vi "Email_With_Log.vi"(0 "recipients":string[](array[string]), 1 "subject ([No Subject])":string="[No Subject]", 2 "message":string, 3 "attachments":T1(array[cluster])) -> (5 "invalid recipients":string[](array[string]), 6 "error out":errorcluster)   [LabVIEW 2016]
uses:
  Globals/Preference_global.vi
  Globals/Constants_global.vi
  <vilib>/Utility/SMTP/NI_SMTPEmail.lvlib
panel:
  out "Number of valid email requests":i32
  # "Image/x-png"
  # "Image/jpeg"
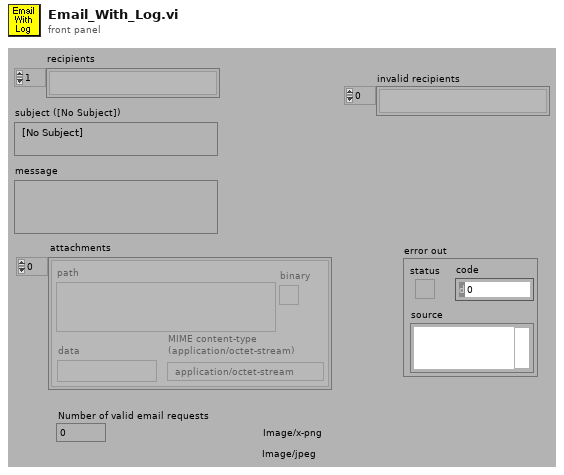
[diagram p1: front panel]
types:
  T1 = cluster{"path":path, "data":string, "binary":bool, "MIME content-type \n(application/octet-stream)":string}[]
  T2 = cluster{"path":path, "data":string, "binary":bool, "MIME content-type \n(application/octet-stream)":string}
  T3 = typedef "SMTPCredentials.ctl" = cluster{"User Name":string, "Password":string, "Reply to Address":string, "From Domain":string}
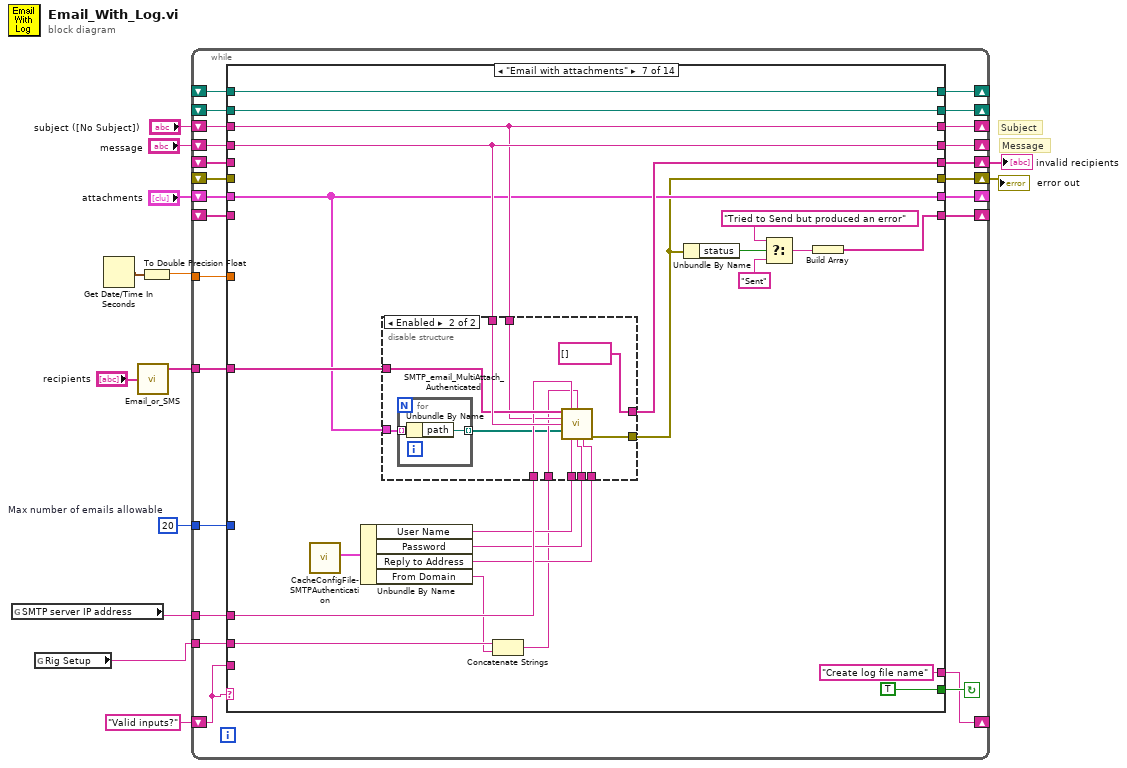
[diagram p0: block diagram]
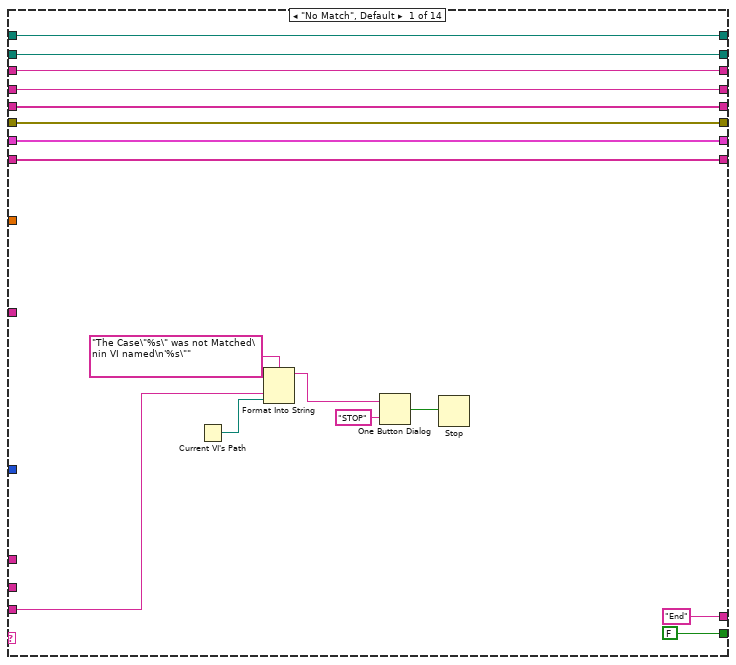
[diagram p2: hidden frame]
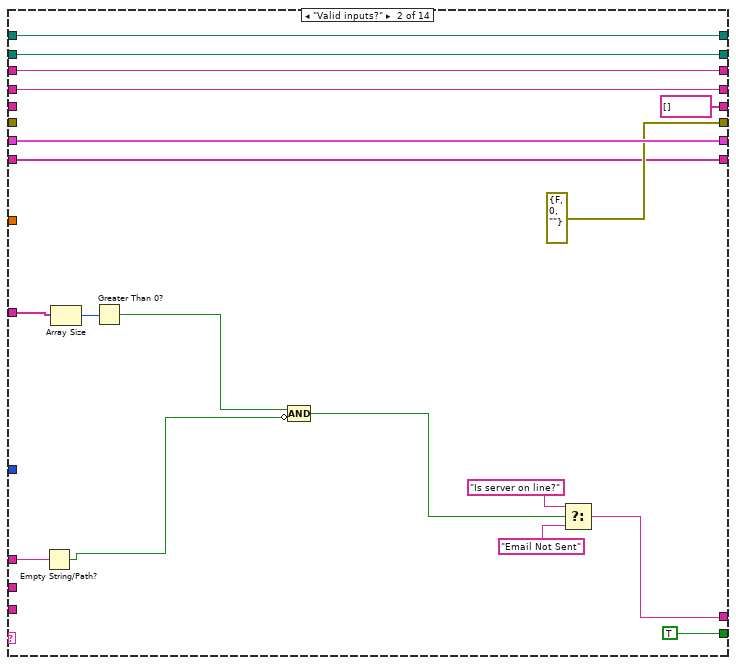
[diagram p3: hidden frame]
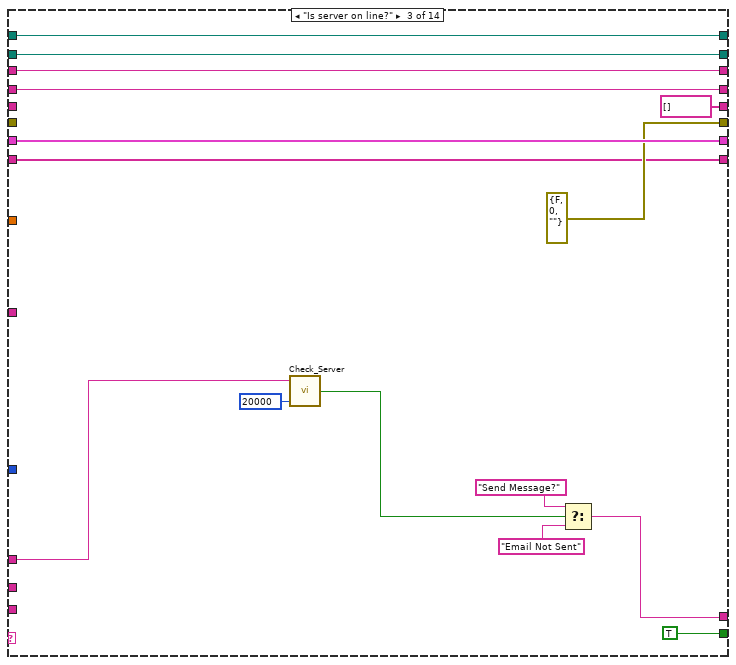
[diagram p4: hidden frame]
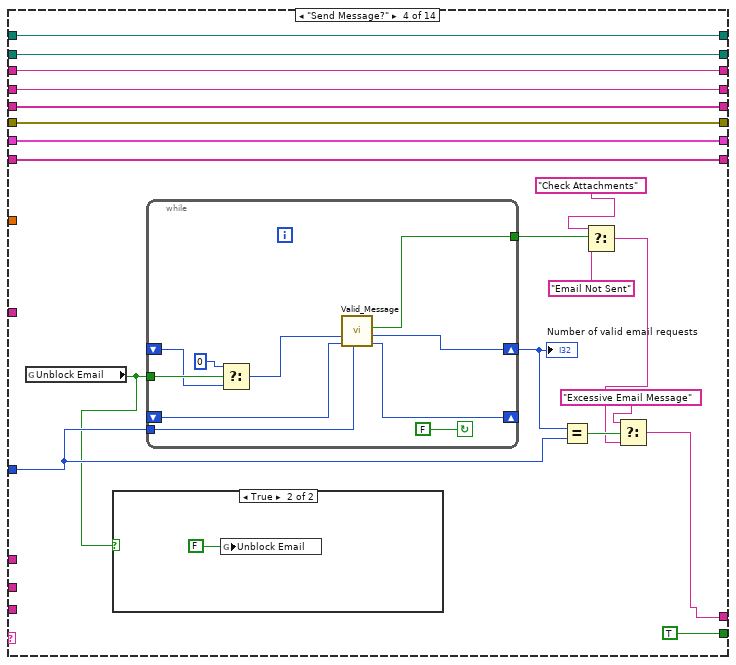
[diagram p5: hidden frame]
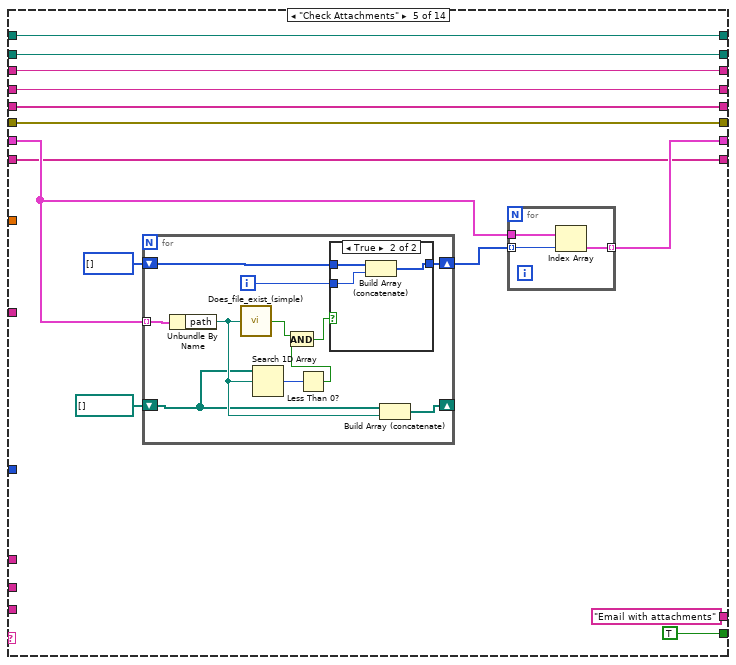
[diagram p7: hidden frame]
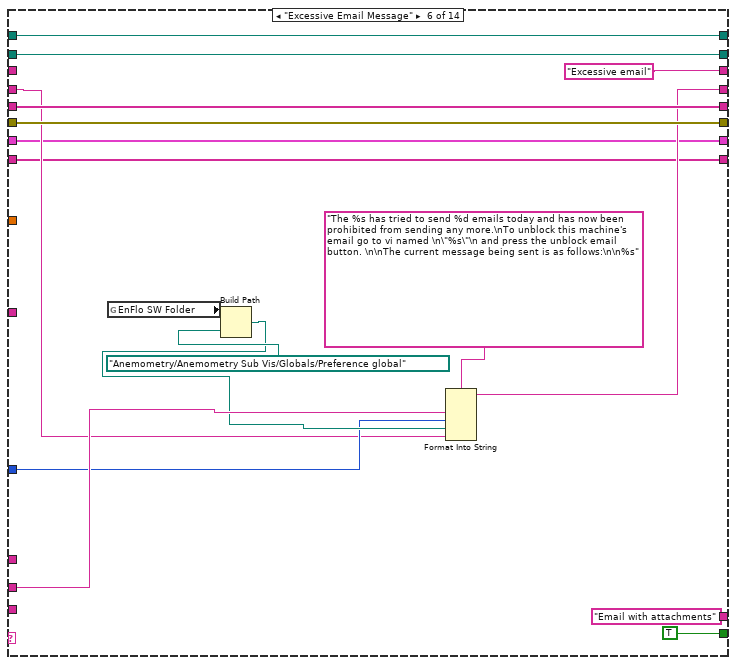
[diagram p9: hidden frame]
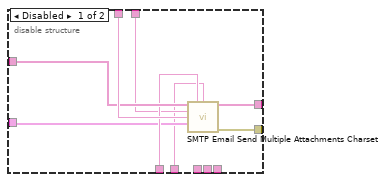
[diagram p10: hidden frame]
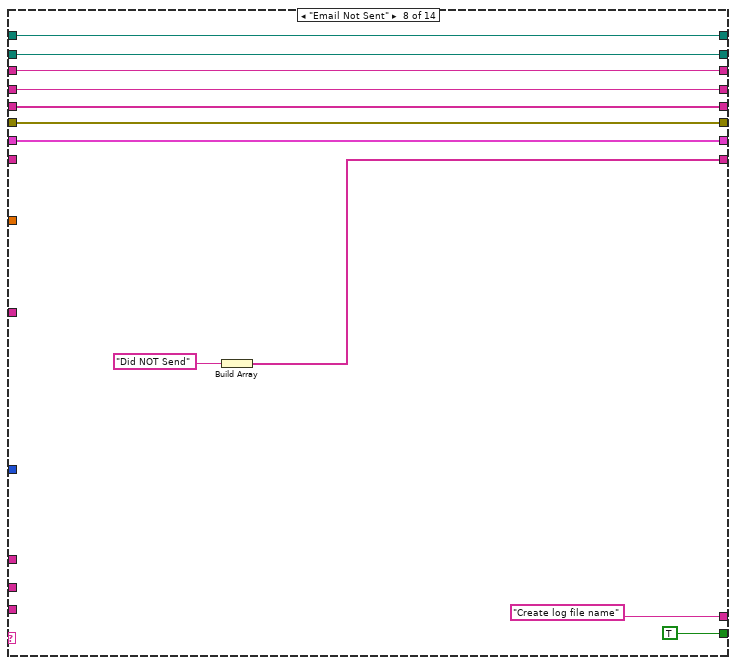
[diagram p11: hidden frame]
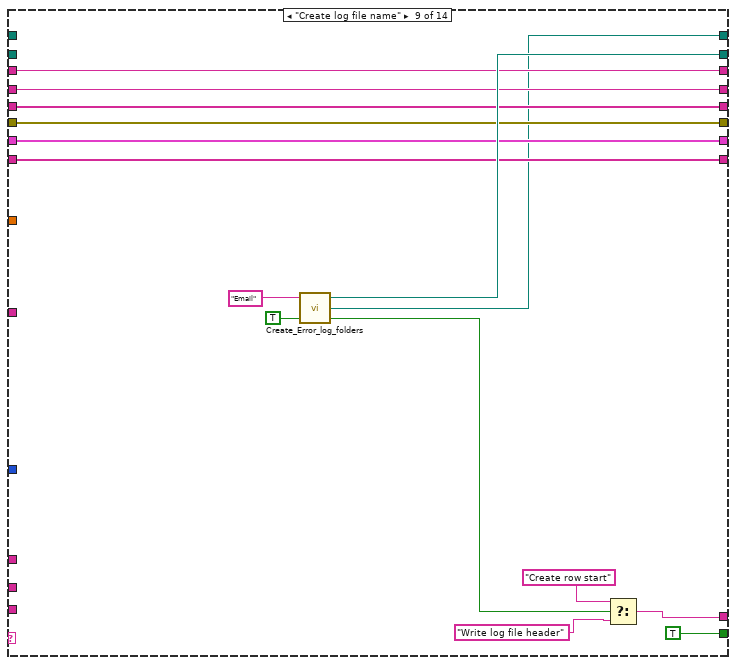
[diagram p12: hidden frame]
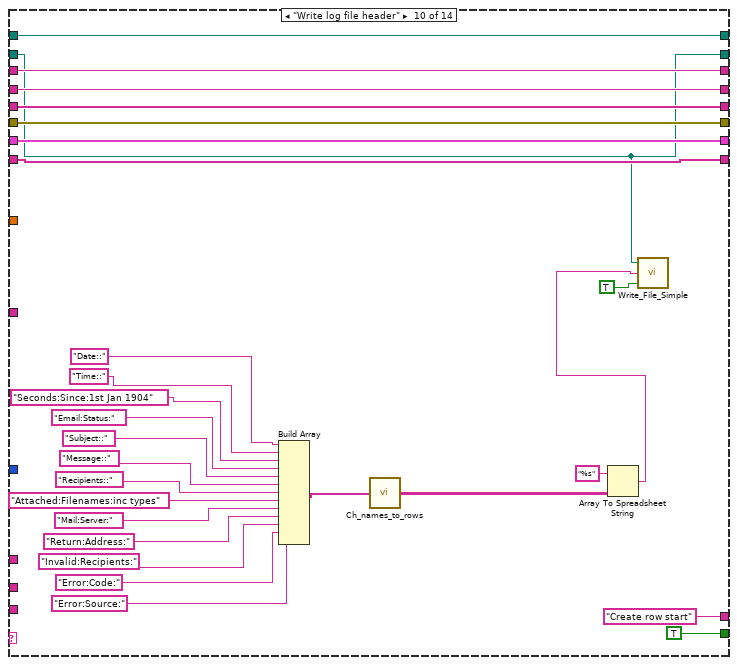
[diagram p13: hidden frame]
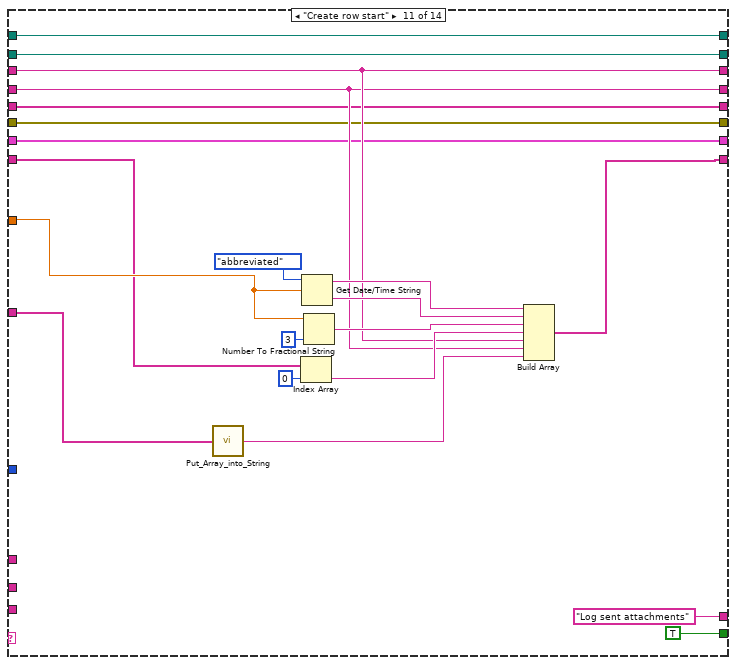
[diagram p14: hidden frame]
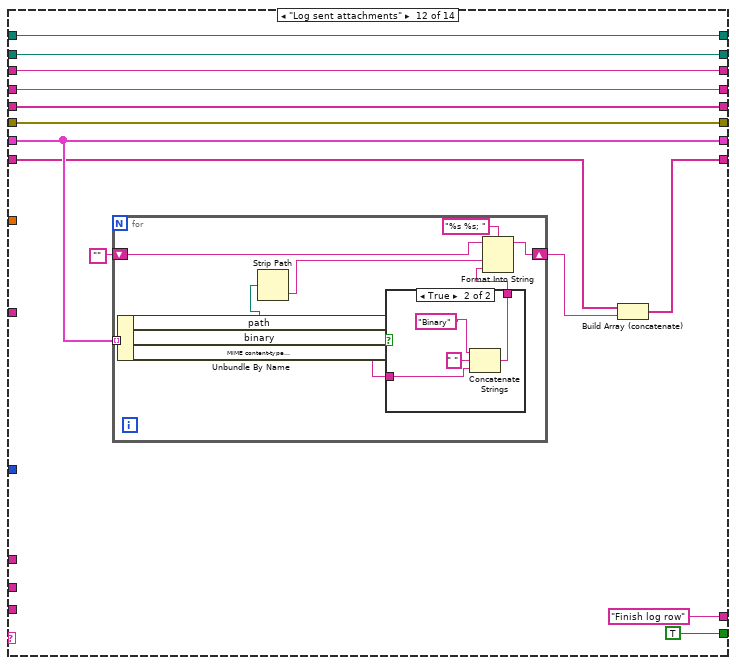
[diagram p15: hidden frame]
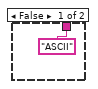
[diagram p16: hidden frame]
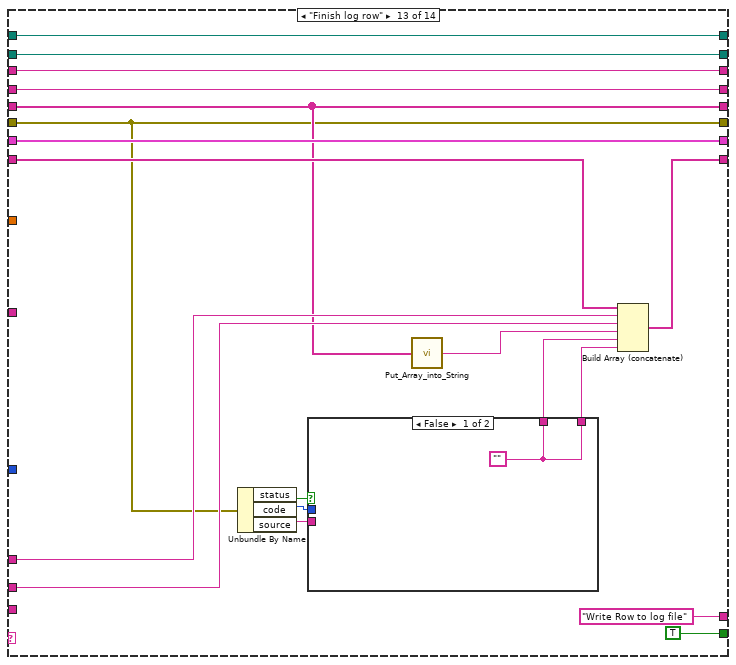
[diagram p17: hidden frame]
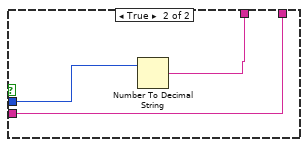
[diagram p18: hidden frame]
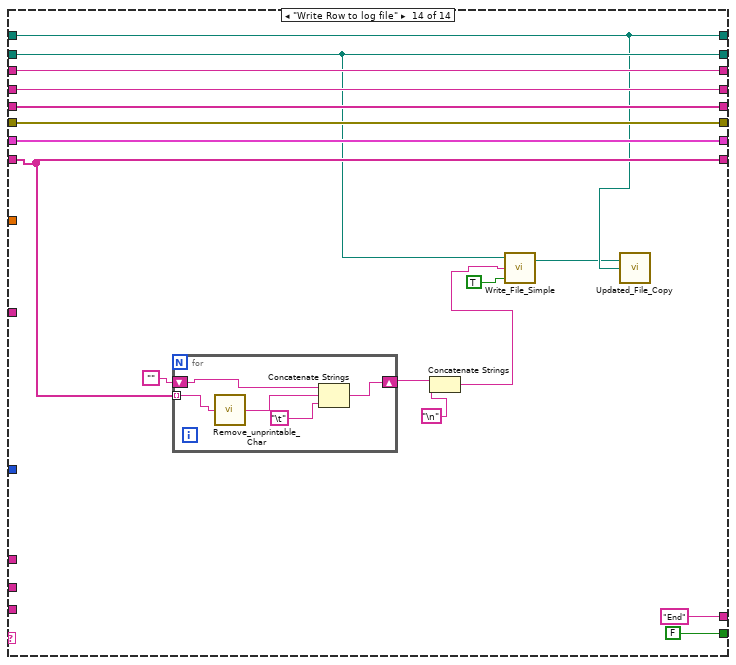
[diagram p19: hidden frame]
diagram:
  w10 = 20  # Max number of emails allowable
  # "Message"
  # "Subject"
  n1 = global read "Preference_global.vi" "SMTP server IP address"() -> (w3:string)
  n2 = global read "Preference_global.vi" "Rig Setup"() -> (w1:string)
  n3 = Get Date/Time In Seconds() -> (seconds since 1Jan1904=w12:timestamp)
  n4 = call "Email_or_SMS.vi"("Email address"="recipients") -> ("Email"=w4:string[])  [unwired: 3 out]
  n5 = To Double Precision Float(number=w12) -> (double precision float=w13:dbl)
  n6 = while {
    tunnel: w13 -> [w35]
    shift-left: "Valid inputs?" -> [w34]
    shift-right: [w36] -> _
    shift-right: [w32] -> _
    shift-left: _ -> [w33]
    tunnel: w10 -> [w31]
    shift-right: [w29] -> _
    shift-left: "subject ([No Subject])" -> [w30]
    shift-right: [w28] -> _
    shift-left: "message" -> [w27]
    shift-right: [w25] -> w8
    shift-left: _ -> [w26]
    shift-right: [w24] -> w2
    shift-left: _ -> [w23]
    tunnel: w1 -> [w22]
    shift-right: [w20] -> _
    shift-left: "attachments" -> [w21]
    tunnel: w4 -> [w19]
    tunnel: w3 -> [w18]
    shift-right: [w17] -> _
    shift-left: _ -> [w16]
    shift-right: [w15] -> _
    shift-left: _ -> [w14]
    stop <- w37 continue-if-true
    n7 = case shown="\"Email with attachments\"" w34 {
      tunnel: [FALSE ("Abort") TRUE ("Abort") TRUE ("Abort") TRUE ("Abort") TRUE ("Abort") TRUE ("Abort") TRUE ("Abort") TRUE ("Abort") TRUE ("status") TRUE TRUE TRUE TRUE FALSE] -> w37
      tunnel: ["End" ("f") w59 w80 w94 "Email with attachments" ("f") "Email with attachments" ("f") "Create log file name" ("f") "Create log file name" ("f") w234 "Create row start" ("f") "Log sent attachments" ("f") "Finish log row" ("f") "Write Row to log file" ("f") "End" ("f")] -> w36
      tunnel: w35 -> [_ _ _ _ _ _ _ _ _ _ w280 _ _ _]
      tunnel: w34 -> [w48 _ _ _ _ _ _ _ _ _ _ _ _ _]
      tunnel: w33 -> [w45 w70 w85 w104 w129 w164 w187 w220 _ w238 w277 w296 w329 w339]
      tunnel: [w45 w70 w85 w104 w129 w164 w187 w220 w231 w238 w277 w296 w329 w339] -> w32
      tunnel: w31 -> [_ _ _ w102 _ w154 _ _ _ _ _ _ _ _]
      tunnel: w30 -> [w44 w69 w84 w101 w128 _ w181 w219 w229 w252 w270 w294 w327 w346]
      tunnel: [w44 w69 w84 w101 w128 "Excessive email" ("Email address") w181 w219 w229 w252 w270 w294 w327 w346] -> w29
      tunnel: [w43 w68 w83 w100 w127 w158 w186 w218 w228 w251 w269 w293 w326 w345] -> w28
      tunnel: w27 -> [w43 w68 w83 w100 w127 w153 w186 w218 w228 w251 w269 w293 w326 w345]
      tunnel: w26 -> [w42 _ _ w99 w126 w163 _ w217 w227 w250 w268 w292 w321 w344]
      tunnel: [w42 string[] [] ("invalid recipients") string[] [] ("invalid recipients") w99 w126 w163 w184 w217 w227 w250 w268 w292 w321 w344] -> w25
      tunnel: [w41 errorcluster {"status"=FALSE, "code"=0, "source"=""} ("error out") errorcluster {"status"=FALSE, "code"=0, "source"=""} ("error out") w98 w125 w162 w179 w216 w226 w249 w267 w291 w319 w343] -> w24
      tunnel: w23 -> [w41 _ _ w98 w125 w162 _ w216 w226 w249 w267 w291 w319 w343]
      tunnel: w22 -> [_ _ _ _ _ w157 w172 _ _ _ _ _ w322 _]
      tunnel: w21 -> [w40 w58 w79 w90 w122 w151 w180 w215 w225 w248 w266 w290 w325 w342]
      tunnel: [w40 w58 w79 w90 w121 w151 w180 w215 w225 w248 w266 w290 w325 w342] -> w20
      tunnel: w19 -> [_ w67 _ _ _ _ w185 _ _ _ w272 _ _ _]
      tunnel: w18 -> [_ w65 w75 _ _ _ w183 _ _ _ _ _ w323 _]
      tunnel: w16 -> [w39 w56 w77 w89 w119 w150 _ _ w224 w241 w276 w287 w324 w341]
      tunnel: [w39 w56 w77 w89 w119 w150 w174 w212 w224 w241 w273 w295 w328 w341] -> w17
      tunnel: [w38 w54 w72 w87 w117 w149 w173 w211 w223 w240 w265 w286 w313 w338] -> w15
      tunnel: w14 -> [w38 w54 w72 w87 w117 w149 w173 w211 _ w240 w265 w286 w313 w338]
      frame "No Match", Default {
        n8 = Current VI's Path() -> (path=w49:path)
        n9 = Format Into String(format string="The Case\"%s\" was not Matched\nin VI named\n'%s\"" ("Format String"), w48, w49) -> (resulting string=w52:string)  [unwired: 2 in, 1 out]
        n10 = One Button Dialog(message=w52, button name ("OK")="STOP") -> (true=w50:bool)
        n11 = Stop(stop? (T)=w50) -> ()
      }
      frame "Valid inputs?" {
        n12 = Empty String/Path?(string/path=w65) -> (empty?=w63:bool)
        n13 = Array Size(array=w67) -> (size(s)=w66:i32)
        n14 = Greater Than 0?(x=w66) -> (x > 0?=w64:bool)
        n15 = Compound Arithmetic op=AND(w64, invert w63) -> (w62:bool)
        n16 = Select(t="Is server on line?" ("f"), s=w62, f="Email Not Sent") -> (s? t:f=w59:string)
      }
      frame "Is server on line?" {
        n17 = call "Check_Server.vi"("timeout ms (60000)"=20000, "address"=w75) -> ("OK"=w74:bool)  [unwired: 3 out]
        n18 = Select(t="Send Message?" ("f"), s=w74, f="Email Not Sent") -> (s? t:f=w80:string)
      }
      frame "Send Message?" {
        n19 = global read "Preference_global.vi" "Unblock Email"() -> (w88:bool)
        n20 = case shown="True" w88 {
          frame False {
          }
          frame True {
            n21 = global write "Preference_global.vi" "Unblock Email"(FALSE ("Unblock Email")) -> ()
          }
        }
        n22 = while {
          tunnel: w88 -> [w111]
          tunnel: w102 -> [w113]
          tunnel: [w114] -> w96
          shift-left: _ -> [w110]
          shift-right: [w112] -> w103
          shift-left: _ -> [w116]
          shift-right: [w115] -> _
          stop <- FALSE continue-if-true
          n23 = Select(t=0, s=w111, f=w110) -> (s? t:f=w109:i32)
          n24 = call "Valid_Message.vi"("Max per day"=w113, "day of month in"=w116, "Number of requests today In"=w109) -> ("day of month out"=w115:i32, "Number of requests today Out"=w112:i32, "Send Message"=w114:bool)  [unwired: 2 in, 4 out]
        }
        "Number of valid email requests" <- w103
        n25 = Equal?(x=w103, y=w102) -> (x = y?=w97:bool)
        n26 = Select(t="Check Attachments", s=w96, f="Email Not Sent") -> (s? t:f=w95:string)
        n27 = Select(t="Excessive Email Message", s=w97, f=w95) -> (s? t:f=w94:string)
      }
      frame "Check Attachments" {
        n28 = for {
          tunnel: w122 -> [w144] mode=indexing
          shift-right: [w141] -> w123
          shift-left: i32[] [] -> [w143]
          shift-right: [w140] -> _
          shift-left: path[] [] -> [w138]
          i -> [w142]
          n29 = Unbundle By Name(w144) -> ("path"=w139:path)
          n30 = call "Does_file_exist_(simple).vi"("Pathname"=w139) -> ("exists?"=w136:bool)
          n31 = Search 1D Array(1D array=w138, element=w139) -> (index of element=w137:i32)  [unwired: 1 out]
          n32 = Less Than 0?(x=w137) -> (x < 0?=w135:bool)
          n33 = And(x=w136, y=w135) -> (x .and. y?=w134:bool)
          n34 = case shown="True" w134 {
            tunnel: w143 -> [w145 w148]
            tunnel: w142 -> [_ w147]
            tunnel: [w145 w146] -> w141
            frame False {
            }
            frame True {
              n35 = Build Array (concatenate)(w148, w147) -> (w146:i32[])
            }
          }
          n36 = Build Array (concatenate)(w138, w139) -> (w140:path[])
        }
        n37 = for {
          tunnel: w123 -> [w133] mode=indexing
          tunnel: w122 -> [w132]
          tunnel: [w131] -> w121 mode=indexing
          n38 = Index Array(array=w132, index=w133) -> (element=w131:T2)
        }
      }
      frame "Excessive Email Message" {
        n39 = global read "Constants_global.vi" "EnFlo SW Folder"() -> (w160:path)
        n40 = Build Path(base path=w160, name or relative path=path "Anemometry/Anemometry Sub Vis/Globals/Preference global") -> (appended path=w156:path)
        n41 = Format Into String(format string="The %s has tried to send %d emails today and has now been prohibited from sending any more.\nTo unblock this machine's email go to vi named \n\"%s\"\n and press the unblock email button. \n\nThe current message being sent is as follows:\n\n%s" ("Format String"), w157, w154, w156, w153) -> (resulting string=w158:string)  [unwired: 2 in, 1 out]
      }
      frame "Email with attachments" {
        n42 = call "CacheConfigFile-SMTPAuthentication.vi"() -> ("Authentication Credentials"=w171:T3)  [unwired: 11 in]
        n43 = Unbundle By Name(w171) -> ("User Name"=w170:string, "Password"=w169:string, "Reply to Address"=w167:string, "From Domain"=w168:string)
        n44 = Concatenate Strings(w172, w168) -> (w166:string)
        n45 = disable-structure shown="Enabled" {
          disable-tunnel: w186 -> [w196 w208]
          disable-tunnel: w185 -> [w195 w207]
          disable-tunnel: [w194 string[] [] ("invalid recipients")] -> w184
          disable-tunnel: w183 -> [w193 w206]
          disable-tunnel: w181 -> [w192 w205]
          disable-tunnel: w180 -> [w191 w204]
          disable-tunnel: [w190 w203] -> w179
          disable-tunnel: w166 -> [w189 w202]
          disable-tunnel: w170 -> [_ w199]
          disable-tunnel: w169 -> [_ w198]
          disable-tunnel: w167 -> [_ w197]
          frame Disabled {
            n46 = call <vilib>:"SMTP Email Send Multiple Attachments Charset.vi"("recipients"=w195, "mail server"=w193, "return address"=w189, "subject ([No Subject])"=w192, "message"=w196, "attachments"=w191) -> ("invalid recipients"=w194:string[], "error out"=w190:errorcluster)  [unwired: 2 in, 6 out]
          }
          frame Enabled {
            n47 = for {
              tunnel: w204 -> [w210] mode=indexing
              tunnel: [w209] -> w201 mode=indexing
              n48 = Unbundle By Name(w210) -> ("path"=w209:path)
            }
            n49 = call "SMTP_email_MultiAttach_Authenticated.vi"("Recipients"=w207, "SMTPServer:Port"=w206, "From Address"=w202, "Subject"=w205, "Message"=w208, "Attachments"=w201, "Username"=w199, "Password"=w198, "Reply-to Address"=w197) -> ("Error Out"=w203:errorcluster)  [unwired: 6 in]
          }
        }
        n50 = Unbundle By Name(w179) -> ("status"=w178:bool)
        n51 = Select(t="Tried to Send but produced an error", s=w178, f="Sent") -> (s? t:f=w175:string)
        n52 = Build Array(w175) -> (w174:string[])
      }
      frame "Email Not Sent" {
        n53 = Build Array("Did NOT Send") -> (w212:string[])
      }
      frame "Create log file name" {
        n54 = call "Create_Error_log_folders.vi"("Per Day Log File?"=TRUE, "Log Filename"="Email" ("Input Element")) -> ("exists?"=w230:bool, "Server copy Location"=w223:path, "Local Log File"=w231:path)  [unwired: 1 in]
        n55 = Select(t="Create row start", s=w230, f="Write log file header") -> (s? t:f=w234:string)
      }
      frame "Write log file header" {
        n56 = Build Array("Date::", "Time::", "Seconds:Since:1st Jan 1904", "Email:Status:", "Subject::", "Message::", "Recipients::", "Attached:Filenames:inc types", "Mail:Server:", "Return:Address:", "Invalid:Recipients:", "Error:Code:", "Error:Source:") -> (w259:string[])
        n57 = call "Ch_names_to_rows.vi"("Channel Names"=w259) -> ("3 Row names"=w258:string[][])
        n58 = Array To Spreadsheet String(array=w258, 3:"%s" ("format string")) -> (spreadsheet string=w237:string)  [unwired: 1 out]
        n59 = call "Write_File_Simple.vi"("append to file? (new file:F)"=TRUE, "character string"=w237, "file path"=w238) -> ()  [unwired: 2 out]
      }
      frame "Create row start" {
        n60 = call "Put_Array_into_String.vi"("String array"=w272) -> ("String Value"=w271:string)
        n61 = Index Array(array=w276, index=0) -> (element=w274:string)
        n62 = Get Date/Time String(date format (0)=enum16{"short", "long", "abbreviated"}."abbreviated", seconds (now)=w280) -> (date string=w284:string, time string=w283:string)  [unwired: 1 out]
        n63 = Number To Fractional String(number=w280, precision (6)=i16 3) -> (F-format string=w279:string)  [unwired: 2 out]
        n64 = Build Array(w284, w283, w279, w274, w270, w269, w271) -> (w273:string[])
      }
      frame "Log sent attachments" {
        n65 = for {
          tunnel: w290 -> [w307] mode=indexing
          shift-right: [w301] -> w288
          shift-left: "" -> [w302]
          n66 = Unbundle By Name(w307) -> ("path"=w306:path, "binary"=w304:bool, "MIME content-type \n(application/octet-stream)"=w303:string)
          n67 = Strip Path(path=w306) -> (name=w305:string)  [unwired: 1 out]
          n68 = case shown="True" w304 {
            tunnel: w303 -> [_ w310]
            tunnel: ["ASCII" w309] -> w300
            frame False {
            }
            frame True {
              n69 = Concatenate Strings("Binary", " " ("string"), w310) -> (w309:string)
            }
          }
          n70 = Format Into String(format string="%s %s; ", initial string=w302, w305, w300) -> (resulting string=w301:string)  [unwired: 1 in, 1 out]
        }
        n71 = Build Array (concatenate)(w287, w288) -> (w295:string[])
      }
      frame "Finish log row" {
        n72 = Unbundle By Name(w319) -> ("status"=w318:bool, "code"=w317:i32, "source"=w316:string)
        n73 = case shown="False" w318 {
          tunnel: w317 -> [_ w334]
          tunnel: w316 -> [_ w335]
          tunnel: [w332 w335] -> w315
          tunnel: [w332 w333] -> w314
          frame False {
            w332 = ""
          }
          frame True {
            n74 = Number To Decimal String(number=w334) -> (decimal integer string=w333:string)  [unwired: 1 out]
          }
        }
        n75 = call "Put_Array_into_String.vi"("String array"=w321) -> ("String Value"=w320:string)
        n76 = Build Array (concatenate)(w324, w323, w322, w320, w314, w315) -> (w328:string[])
      }
      frame "Write Row to log file" {
        n77 = for {
          shift-right: [w355] -> w347
          shift-left: "" -> [w356]
          tunnel: w341 -> [w353] mode=indexing
          n78 = call "Remove_unprintable_Char.vi"("Input String"=w353) -> ("Output String"=w352:string)
          n79 = Concatenate Strings(w356, w352, "\t") -> (w355:string)
        }
        n80 = Concatenate Strings(w347, "\n") -> (w340:string)
        n81 = call "Write_File_Simple.vi"("append to file? (new file:F)"=TRUE, "character string"=w340, "file path"=w339) -> ("file path Out"=w336:path)  [unwired: 1 out]
        n82 = call "Updated_File_Copy.vi"("Target Path"=w338, "Source Path"=w336) -> ()  [unwired: 2 out]
      }
    }
  }
  "invalid recipients" <- w8
  "error out" <- w2
